vi "Obtain Request Events.vi"(8 "error in":errorcluster, 10 "Create New? (F)":bool) -> (0 "error out":errorcluster, 2 "Motor Request Events":T1)   [LabVIEW 2022 SP3, in "Motor.lvlib"]
doc: "This VI Obtains/Creates the Requests events that will be used for other modules to communicate with the module that owns this VI. These Requests events will be accessed only via Public API methods for this module.\n\n<b>NOTE</b>: The contents of this VI are automatically generated and modified by the <b>Tools > DQMH Consortium > DQMH</b> utilities. Consider using those utilities instead of making your own modifications to this VI.\n_____\nBased on DQMH Project Template 7.0.1.1316."
uses:
  Motor.lvlib
  Request Events--cluster.ctl
  Stop Argument--cluster.ctl
  Show Panel Argument--cluster.ctl
  Hide Panel Argument--cluster.ctl
  Get Module Execution Status Argument--cluster.ctl
  Show Diagram Argument--cluster.ctl
panel:
  # "NOTE: The contents of this VI are automatically generated and modified by the Tools > DQMH Consortium > DQMH utilities. Consider using those utilities instead of making your own modifications to this VI."
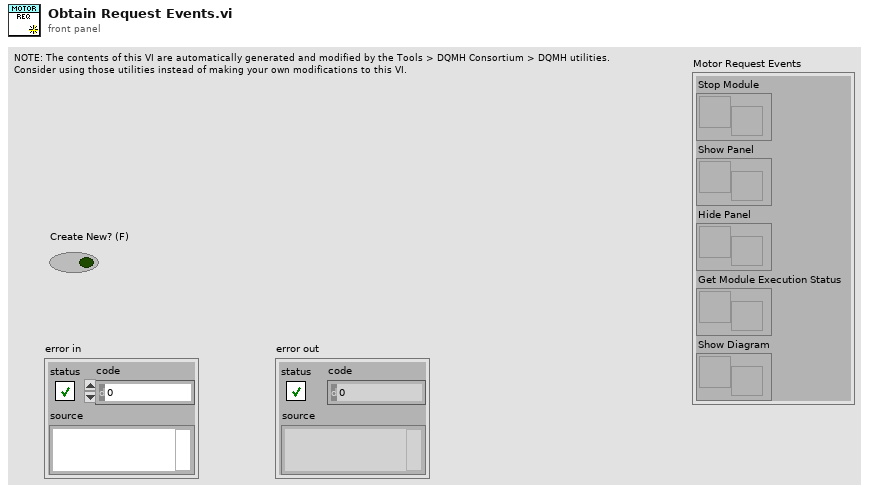
[diagram p1: front panel]
types:
  T1 = typedef "Motor.lvlib/Request Events--cluster.ctl" = cluster{"Stop Module":refnum<user-event>, "Show Panel":refnum<user-event>, "Hide Panel":refnum<user-event>, "Get Module Execution Status":refnum<user-event>, "Show Diagram":refnum<user-event>}
  T2 = typedef "Motor.lvlib/Hide Panel Argument--cluster.ctl" = cluster{"Hide Panel?":bool}
  T3 = typedef "Motor.lvlib/Show Panel Argument--cluster.ctl" = cluster{"Show Panel?":bool}
  T4 = typedef "Motor.lvlib/Show Diagram Argument--cluster.ctl" = cluster{"Debug?":bool}
  T5 = typedef "Motor.lvlib/Get Module Execution Status Argument--cluster.ctl" = cluster{"Running?":bool}
  T6 = typedef "Motor.lvlib/Stop Argument--cluster.ctl" = cluster{"Origin":string, "Exit via Stop Module Req?":bool, "Wait for Module to stop?":bool}
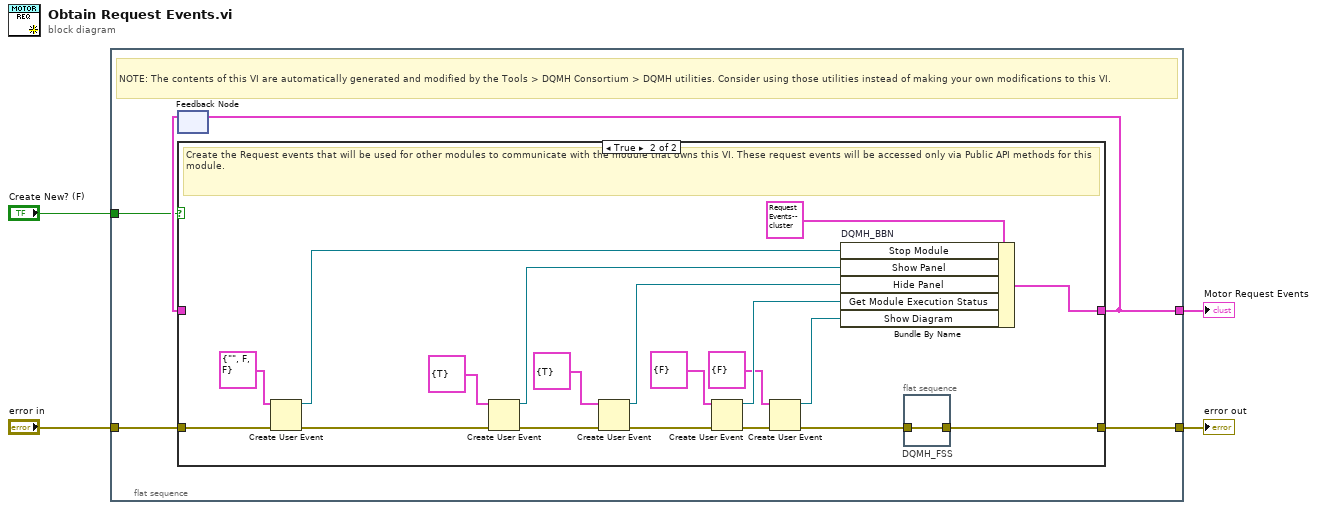
[diagram p0: block diagram]
diagram:
  n1 = flat-sequence {
    tunnel: [w9] -> w4
    tunnel: "error in" -> [w8]
    tunnel: [w6] -> w2
    tunnel: "Create New? (F)" -> [w5]
    frame #0 {
      # "NOTE: The contents of this VI are automatically generated and modified by the Tools > DQMH Consortium > DQMH utilities. Consider using those utilities instead of making your own modifications to this VI."
      n2 = feedback #1() -> (w7:T1)  [unwired: 1 in]
      n3 = case shown="True" w5 {
        tunnel: [w10 w20] -> w9
        tunnel: w8 -> [w10 w30]
        tunnel: [w11 w27] -> w6
        tunnel: w7 -> [w11 _]
        frame False {
          # "Obtain the Request events that were created in a previous call to this VI."
        }
        frame True {
          # "Create the Request events that will be used for other modules to communicate with the module that owns this VI. These request events will be accessed only via Public API methods for this module."
          n4 = Create User Event(user event datatype=T6 {"Origin"="", "Exit via Stop Module Req?"=FALSE, "Wait for Module to stop?"=FALSE} ("Stop Argument"), error in=w30) -> (user event=w28:refnum<user-event>, error out=w25:errorcluster)
          n5 = Create User Event(user event datatype=T3 {"Show Panel?"=TRUE} ("Show Panel Argument"), error in=w25) -> (user event=w24:refnum<user-event>, error out=w23:errorcluster)
          n6 = Create User Event(user event datatype=T2 {"Hide Panel?"=TRUE} ("Hide Panel Argument"), error in=w23) -> (user event=w22:refnum<user-event>, error out=w21:errorcluster)
          n7 = Create User Event(user event datatype=T5 {"Running?"=FALSE} ("Get Module Execution Status Argument"), error in=w21) -> (user event=w18:refnum<user-event>, error out=w19:errorcluster)
          n8 = Create User Event(user event datatype=T4 {"Debug?"=FALSE} ("Show Diagram Argument"), error in=w19) -> (user event=w15:refnum<user-event>, error out=w16:errorcluster)
          n9 = Bundle By Name "DQMH_BBN"(cluster=T1 {"Stop Module"=refnum, "Show Panel"=refnum, "Hide Panel"=refnum, "Get Module Execution Status"=refnum, "Show Diagram"=refnum} ("output cluster"), "Stop Module"=w28, "Show Panel"=w24, "Hide Panel"=w22, "Get Module Execution Status"=w18, "Show Diagram"=w15) -> (w27:T1)
          n10 = flat-sequence "DQMH_FSS" {
            tunnel: w16 -> [w31]
            tunnel: [w31] -> w20
            frame #0 {
            }
          }
        }
      }
      n11 = feedback-in #1(w6) -> ()
    }
  }
  "Motor Request Events" <- w2
  "error out" <- w4
